vi "Maintain Heading.vi"(9 "PID gains":T1={"proportional gain (Kc)"=1.0, "integral time (Ti, min)"=0.01, "derivative time (Td, min)"=0.0} {"derivative time (Td, min)" format="%.3f"; "integral time (Ti, min)" format="%.3f"; "proportional gain (Kc)" format="%.3f"}, 10 "NavX Yaw":dbl, 11 "Raw Driver Joystick X2":dbl) -> (3 "Driver Joystick X2":dbl)   [LabVIEW 2014]
uses:
  <vilib>/Rock Robotics/WPI/DriverStation/WPI_DriverStationRobotMode2.ctl
  Begin/Global Variables.vi
  <vilib>/addons/control/pid/pid.llb/PID (DBL).vi
  <vilib>/addons/control/pid/NI_PID_pid.lvlib
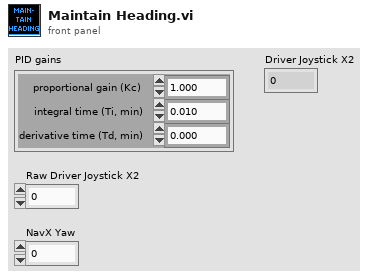
[diagram p1: front panel]
types:
  T1 = cluster{"proportional gain (Kc)":dbl, "integral time (Ti, min)":dbl, "derivative time (Td, min)":dbl}
  T2 = typedef "WPI_DriverStationRobotMode2.ctl" = enum16{"Autonomous Disabled", "Autonomous Enabled", "Teleop Disabled", "Teleop Enabled", "Disconnected", "Finish", "Test Disabled", "Test Enabled", "Emergency Stopped"}
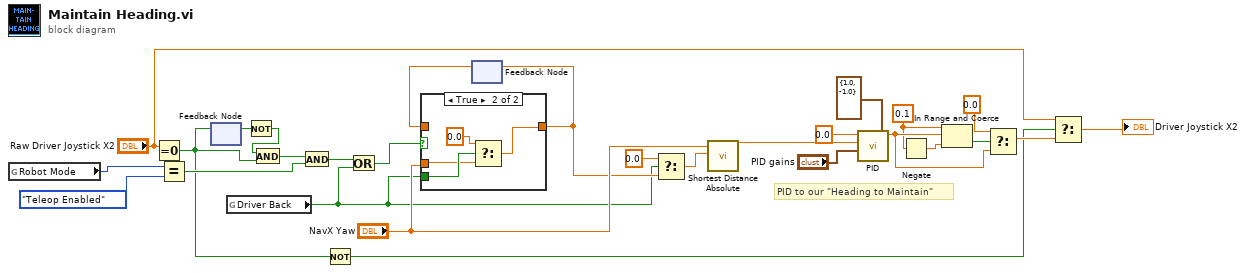
[diagram p0: block diagram]
diagram:
  w20 = 0.1 ("Value to Deadband (default of 0.1)")
  # "PID to our \"Heading to Maintain\""
  n1 = global read "Global Variables.vi" "Robot Mode"() -> (w2:T2)
  n2 = Equal To 0?(x="Raw Driver Joystick X2") -> (x = 0?=w7:bool)
  n3 = Equal?(x=w2, y=WPI_DriverStationRobotMode2."Teleop Enabled") -> (x = y?=w25:bool)
  n4 = feedback #1() -> (w9:bool)  [unwired: 1 in]
  n5 = feedback-in #1(w7) -> ()
  n6 = global read "Global Variables.vi" "Driver Back"() -> (w3:bool)
  n7 = Not(x=w9) -> (.not. x?=w8:bool)
  n8 = And(x=w8, y=w7) -> (x .and. y?=w23:bool)
  n9 = And(x=w23, y=w25) -> (x .and. y?=w26:bool)
  n10 = Not(x=w7) -> (.not. x?=w6:bool)
  n11 = Or(x=w26, y=w3) -> (x .or. y?=w27:bool)
  n12 = feedback #2() -> (w4:dbl)  [unwired: 1 in]
  n13 = case shown="True" w27 {
    tunnel: w3 -> [_ w33]
    tunnel: "NavX Yaw" -> [_ w31]
    tunnel: [w29 w30] -> w5
    tunnel: w4 -> [w29 _]
    frame False {
    }
    frame True {
      n14 = Select(t=0.0, s=w33, f=w31) -> (s? t:f=w30:dbl)
    }
  }
  n15 = feedback-in #2(w5) -> ()
  n16 = Select(t=0.0, s=w3, f=w5) -> (s? t:f=w12:dbl)
  n17 = call "Shortest Distance Absolute.vi"("current"=w12, "target"="NavX Yaw") -> ("shortest angle"=w16:dbl)  [unwired: 9 in]
  n18 = call-poly <vilib>:"PID.vi"("output range"=cluster{"output high":dbl, "output low":dbl} {"output high"=1.0, "output low"=-1.0}, "PID gains"="PID gains", "process variable"=w16, "setpoint"=0.0) -> ("output"=w22:dbl)  [unwired: 6 in, 1 out]
  n19 = Negate(x=w20) -> (-x=w21:dbl)
  n20 = In Range and Coerce(upper limit=w20, x=w22, lower limit=w21) -> (In Range?=w19:bool)  [unwired: 1 out]
  n21 = Select(t=0.0, s=w19, f=w22) -> (s? t:f=w28:dbl)
  n22 = Select(t="Raw Driver Joystick X2", s=w6, f=w28) -> (s? t:f=→"Driver Joystick X2":dbl)
